vi "Convert_Fault.vi"(0 "ERD Data Out":T2[](array[typedef]) {"ERD Number" format="%.0x"}, 11 "Error In":errorcluster) -> (3 "Fault Entry 1":T1, 4 "Fault Entry 2":T1, 6 "Fault Entry 3":T1, 8 "Fault Entry 4":T1, 10 "Fault Entry 5":T1, 15 "Error Out":errorcluster)   [LabVIEW 2014]
uses:
  Utility/Labview GEA2 Toolkit v2.1/type defs/ERD Read Data Out.ctl
  type defs/Fault_Info.ctl
  Utility/Labview GEA2 Toolkit v2.1/library/GEA2_Toolkit.lvlib
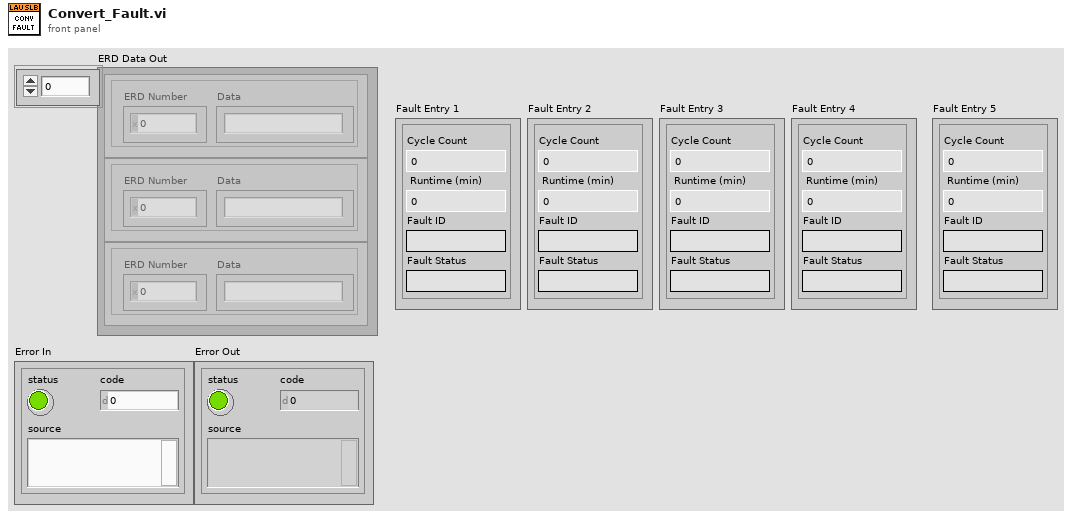
[diagram p1: front panel]
types:
  T1 = typedef "Fault_Info.ctl" = cluster{"Cycle Count":u32, " Runtime (min) ":u32, "Fault Status":string, "Fault ID":string}
  T2 = typedef "GEA2_Toolkit.lvlib/ERD Read Data Out.ctl" = cluster{"ERD Number":u16, "Data":string}
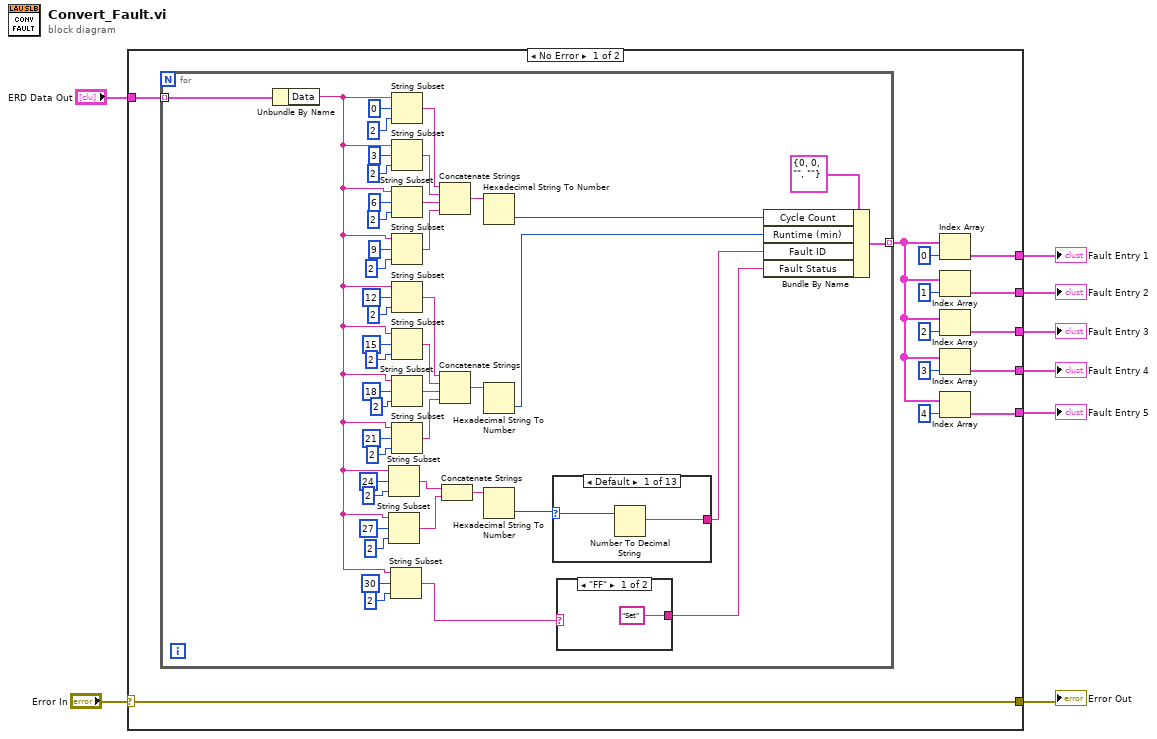
[diagram p0: block diagram]
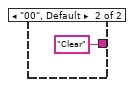
[diagram p2: hidden frame]
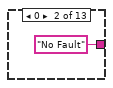
[diagram p3: hidden frame]
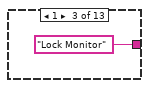
[diagram p4: hidden frame]
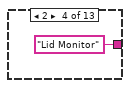
[diagram p5: hidden frame]
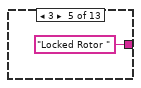
[diagram p6: hidden frame]
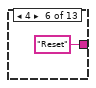
[diagram p7: hidden frame]
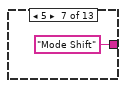
[diagram p8: hidden frame]
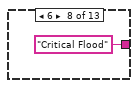
[diagram p9: hidden frame]
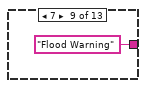
[diagram p10: hidden frame]
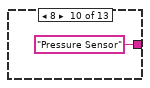
[diagram p11: hidden frame]
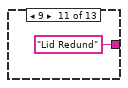
[diagram p12: hidden frame]
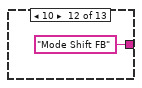
[diagram p13: hidden frame]
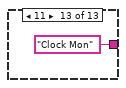
[diagram p14: hidden frame]
diagram:
  n1 = case shown="No Error" "Error In" {
    selector: "Error In" -> [w20 w83]
    tunnel: [w20 w83] -> w7
    tunnel: "ERD Data Out" -> [w21 _]
    tunnel: [w13 _] -> w5
    tunnel: [w12 _] -> w4
    tunnel: [w11 _] -> w3
    tunnel: [w10 _] -> w2
    tunnel: [w9 _] -> w1
    frame No Error {
      n2 = for {
        tunnel: w21 -> [w23] mode=indexing
        tunnel: [w22] -> w14 mode=indexing
        n3 = Unbundle By Name(w23) -> ("Data"=w37:string)
        n4 = String Subset(string=w37, offset (0)=24, length (rest)=2 ("length (rest)")) -> (substring=w45:string)
        n5 = String Subset(string=w37, offset (0)=27, length (rest)=2 ("length (rest)")) -> (substring=w44:string)
        n6 = String Subset(string=w37, offset (0)=30, length (rest)=2 ("length (rest)")) -> (substring=w25:string)
        n7 = String Subset(string=w37, offset (0)=0, length (rest)=2 ("length (rest)")) -> (substring=w62:string)
        n8 = String Subset(string=w37, offset (0)=3, length (rest)=2 ("length (rest)")) -> (substring=w61:string)
        n9 = String Subset(string=w37, offset (0)=6, length (rest)=2 ("length (rest)")) -> (substring=w60:string)
        n10 = String Subset(string=w37, offset (0)=9, length (rest)=2 ("length (rest)")) -> (substring=w59:string)
        n11 = String Subset(string=w37, offset (0)=12, length (rest)=2 ("length (rest)")) -> (substring=w52:string)
        n12 = String Subset(string=w37, offset (0)=15, length (rest)=2 ("length (rest)")) -> (substring=w53:string)
        n13 = String Subset(string=w37, offset (0)=18, length (rest)=2 ("length (rest)")) -> (substring=w54:string)
        n14 = String Subset(string=w37, offset (0)=21, length (rest)=2 ("length (rest)")) -> (substring=w55:string)
        n15 = Concatenate Strings(w62, w61, w60, w59) -> (w58:string)
        n16 = Concatenate Strings(w52, w53, w54, w55) -> (w56:string)
        n17 = Concatenate Strings(w45, w44) -> (w43:string)
        n18 = Hexadecimal String To Number(string=w58) -> (number=w57:u32)  [unwired: 2 in, 1 out]
        n19 = Hexadecimal String To Number(string=w56) -> (number=w39:u32)  [unwired: 2 in, 1 out]
        n20 = Hexadecimal String To Number(string=w43) -> (number=w42:u32)  [unwired: 2 in, 1 out]
        n21 = case shown="Default" w42 {
          selector: w42 -> [w70 _ _ _ _ _ _ _ _ _ _ _ _]
          tunnel: [w69 "No Fault" "Lock Monitor" "Lid Monitor" "Locked Rotor " "Reset" "Mode Shift" "Critical Flood" "Flood Warning" "Pressure Sensor" "Lid Redund" "Mode Shift FB" "Clock Mon"] -> w41
          frame Default {
            n22 = Number To Decimal String(number=w70) -> (decimal integer string=w69:string)  [unwired: 1 in]
          }
          frame 0 {
          }
          frame 1 {
          }
          frame 2 {
          }
          frame 3 {
          }
          frame 4 {
          }
          frame 5 {
          }
          frame 6 {
          }
          frame 7 {
          }
          frame 8 {
          }
          frame 9 {
          }
          frame 10 {
          }
          frame 11 {
          }
        }
        n23 = case shown="\"FF\"" w25 {
          tunnel: ["Set" "Clear"] -> w24
          frame "FF" {
          }
          frame "00", Default {
          }
        }
        n24 = Bundle By Name(cluster=T1 {"Cycle Count"=0, " Runtime (min) "=0, "Fault Status"="", "Fault ID"=""} ("Fault Entry 2"), "Cycle Count"=w57, "Runtime (min)"=w39, "Fault ID"=w41, "Fault Status"=w24) -> (w22:T1)
      }
      n25 = Index Array(array=w14, index=0) -> (element=w13:T1)
      n26 = Index Array(array=w14, index=1) -> (element=w12:T1)
      n27 = Index Array(array=w14, index=2) -> (element=w11:T1)
      n28 = Index Array(array=w14, index=3) -> (element=w10:T1)
      n29 = Index Array(array=w14, index=4) -> (element=w9:T1)
    }
    frame Error {
    }
  }
  "Error Out" <- w7
  "Fault Entry 2" <- w4
  "Fault Entry 3" <- w3
  "Fault Entry 4" <- w2
  "Fault Entry 5" <- w1
  "Fault Entry 1" <- w5
